vi "Begin.vi"() -> (0 "error out":errorcluster)   [LabVIEW 2013]
doc: "Called before other user functions, this VI is expected to open initial I/O refnums, load in file data, and do all program initialization. Notice that the <B>error out</B> terminal is simply used for data flow. Wiring it to other structures or subVIs ensures that this VI runs first."
uses:
  <vilib>/Rock Robotics/WPI/SafetyOutput/WPI_SafetyOutputConfigMenu.ctl
  <vilib>/Rock Robotics/WPI/DriverStation/WPI_DriverStationRobotMode2.ctl
  <vilib>/Rock Robotics/WPI/Joystick/WPI_JoystickDeviceEnum.ctl
  <vilib>/Rock Robotics/SystemInterfaces/DIO/FPGA_DIOPWMChannel.ctl
  <vilib>/Rock Robotics/SystemInterfaces/DIO/FPGA_DIOChannel.ctl
  <vilib>/Rock Robotics/SystemInterfaces/DIO/FPGA_DIORelayChannel.ctl
  <vilib>/Rock Robotics/SystemInterfaces/Typedef/FPGA_TypedefDigitalModule.ctl
  <vilib>/Rock Robotics/WPI/Camera/WPI_CameraImageSize.ctl
  <vilib>/Rock Robotics/WPI/Camera/WPI_CameraFrameRate.ctl
  <vilib>/Rock Robotics/WPI/Camera/WPI_CameraWhite Balance Values.ctl
  <vilib>/Rock Robotics/WPI/Camera/WPI_CameraExposure Values.ctl
  <vilib>/Rock Robotics/WPI/Solenoid/WPI_SolenoidChannel.ctl
  <vilib>/Rock Robotics/SystemInterfaces/AI/FPGA_AIChannel.ctl
  <vilib>/Rock Robotics/SystemInterfaces/Typedef/FPGA_TypedefAnalogModule.ctl
  Robot Global Data.vi
  <vilib>/Rock Robotics/WPI/MotorControl/WPI_MotorControlOpen Talon.vi
  <vilib>/Rock Robotics/WPI/Solenoid/WPI_SolenoidOpenDouble.vi
  <vilib>/Rock Robotics/WPI/RobotDrive/WPI_RobotDriveOpen4MotorWithTalon.vi
  <vilib>/Rock Robotics/WPI/Compressor/WPI_CompressorGetSetRefNum.vi
panel:
  out "Boolean Array":bool[](array[boolean])
  in  "Dashbord/Constant":bool
  out "error out 3":errorcluster
  out "error out 2":errorcluster
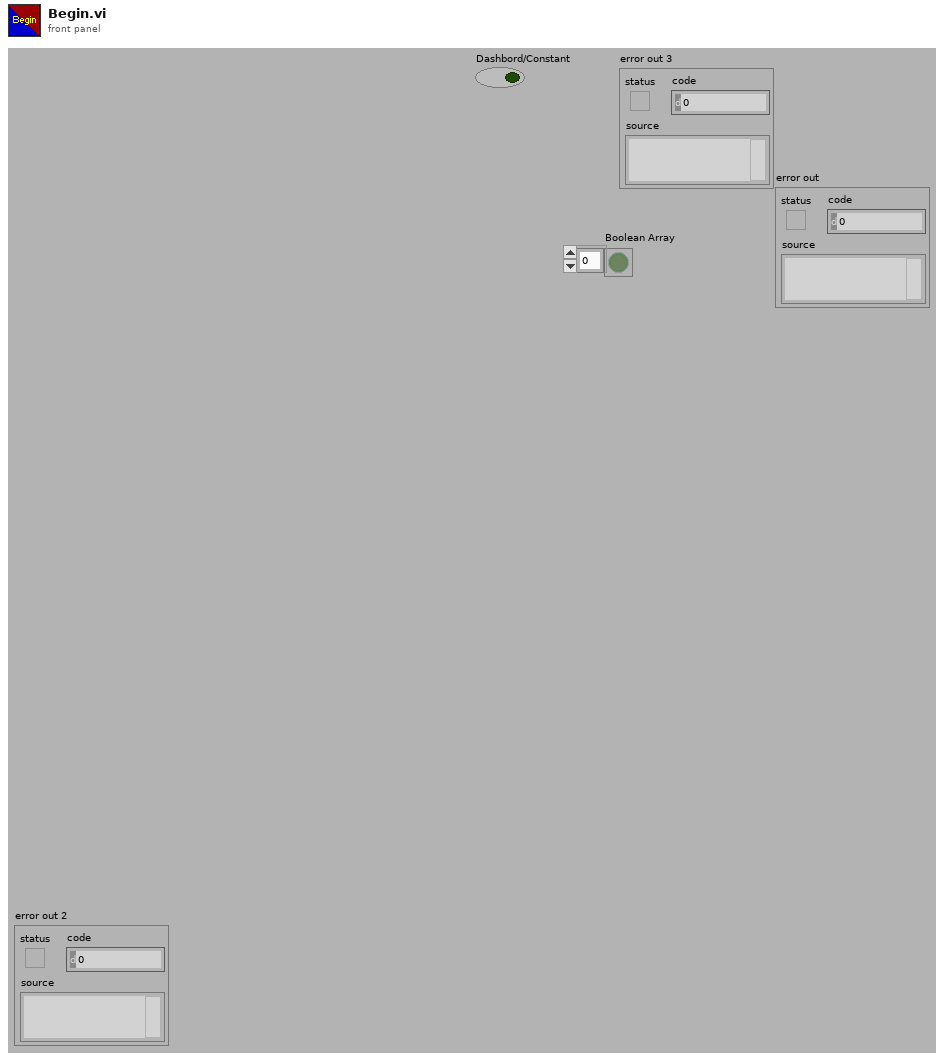
[diagram p1: front panel]
types:
  T1 = typedef "FPGA_TypedefAnalogModule.ctl" = enum16{"Analog Module 1", "Analog Module 2"}
  T2 = typedef "FPGA_AIChannel.ctl" = enum8{"AI 1", "AI 2", "AI 3", "AI 4", "AI 5", "AI 6", "AI 7", "AI 8", "Invalid"}
  T3 = typedef "WPI_SolenoidChannel.ctl" = enum8{"Solenoid 1", "Solenoid 2", "Solenoid 3", "Solenoid 4", "Solenoid 5", "Solenoid 6", "Solenoid 7", "Solenoid 8", "Invalid"}
  T4 = typedef "FPGA_TypedefDigitalModule.ctl" = enum16{"Digital Module 1", "Digital Module 2"}
  T5 = typedef "WPI_CameraExposure Values.ctl" = enum16{"Auto", "Flicker-free 50 Hz", "Flicker-free 60 Hz", "Hold current"}
  T6 = typedef "WPI_CameraWhite Balance Values.ctl" = enum16{"Auto", "Fixed indoor", "Fixed outdoor 1", "Fixed outdoor 2", "Fixed fluorescent 1", "Fixed fluorescent 2", "Hold current"}
  T7 = typedef "WPI_CameraFrameRate.ctl" = u32
  T8 = typedef "WPI_CameraImageSize.ctl" = enum16{"640x480", "320x240", "160x120"}
  T9 = typedef "FPGA_DIOChannel.ctl" = enum8{"DIO 1", "DIO 2", "DIO 3", "DIO 4", "DIO 5", "DIO 6", "DIO 7", "DIO 8", "DIO 9", "DIO 10", "DIO 11", "DIO 12", "DIO 13", "DIO 14", "Invalid"}
  T10 = typedef "FPGA_DIORelayChannel.ctl" = enum8{"Relay 1", "Relay 2", "Relay 3", "Relay 4", "Relay 5", "Relay 6", "Relay 7", "Relay 8", "Invalid"}
  T11 = typedef "WPI_JoystickDeviceEnum.ctl" = enum16{"USB 1", "USB 2", "USB 3", "USB 4", "Kinect 1", "Kinect 2"}
  T12 = typedef "FPGA_DIOPWMChannel.ctl" = enum8{"PWM 1", "PWM 2", "PWM 3", "PWM 4", "PWM 5", "PWM 6", "PWM 7", "PWM 8", "PWM 9", "PWM 10", "Invalid"}
  T13 = typedef "WPI_DriverStationRobotMode2.ctl" = enum16{"Autonomous Disabled", "Autonomous Enabled", "Teleop Disabled", "Teleop Enabled", "Timeout", "Finish", "Test Disabled", "Test Enabled"}
  T14 = typedef "WPI_SafetyOutputConfigMenu.ctl" = enum16{"Enable", "Disable"}
  T15 = cluster{"Boolean Array[0]":bool, "Boolean Array[1]":bool, "Boolean Array[2]":bool, "Boolean Array[3]":bool, "Boolean Array[4]":bool, "Boolean Array[5]":bool, "Boolean Array[6]":bool, "Boolean Array[7]":bool, "Boolean Array[8]":bool}
  T16 = typedef "WPI_MotorControlDeviceRef.ctl" = cluster{"DeviceStatus":errorcluster, "Type":enum16{"PWM", "CAN"}, "PWM":cluster{"Digital Module":T4, "PWM Channel":T12, "DeadBand":T17}, "CAN":cluster{"Device Number":u8, "Control Mode":T18, "Semaphore":T19, "Max Vout":dbl}, "Invert":bool, "TransformRef":T20, "InvTransformRef":T20}
  T17 = typedef "WPI_PWMDeadband.ctl" = cluster{"Name":string, "maxPositivePwm":i32, "minPositivePwm":i32, "centerPwm":i32, "maxNegativePwm":i32, "minNegativePwm":i32, "angularRange":u16}
  T18 = typedef "WPI_CANJaguar_ControlMode.ctl" = enum8{"Percent VBus", "Current", "Speed", "Position", "Voltage"}
  T19 = typedef "Semaphore RefNum" = refnum<k1>
  T20 = typedef "WPI_PWMTransform_ConPane.ctl" = refnum<vi>
  T21 = typedef "WPI_RobotDriveDevRef.ctl" = cluster{"DevStatus":errorcluster, "Motors[]":T16[], "Square Inputs":bool, "Max Output":dbl, "Isochronous":bool}
  T22 = typedef "WPI_CompressorDevRef.ctl" = cluster{"DevStatus":errorcluster, "DigitalInputDevRef":T23, "RelayDevRef":T24}
  T23 = typedef "WPI_DigitalInputDevRef.ctl" = cluster{"DevStatus":errorcluster, "DIO Channel":T9, "Digital Module":T4}
  T24 = typedef "WPI_RelayDevRef.ctl" = cluster{"DevStatus":errorcluster, "Relay Channel":T10, "Digital Module":T4, "Relay Direction":T25}
  T25 = typedef "WPI_RelayDirection.ctl" = enum16{"Both directions", "Forward only", "Reverse only"}
  T26 = typedef "WPI_CameraDevRef.ctl" = cluster{"Camera Address":string, "CameraStatus":errorcluster, "Acquire Image Notifier":refnum<notifier>}
  T27 = typedef "WPI_SolenoidDevRef.ctl" = cluster{"DevStatus":errorcluster, "Solenoid Module":T28, "Forward Solenoid Channel":T3, "Reverse Solenoid Channel":T3}
  T28 = typedef "FPGA_TypedefSolenoidModule.ctl" = enum16{"Solenoid Module 1", "Solenoid Module 2"}
  T29 = typedef "WPI_JoystickDevRef.ctl" = cluster{"Device":T11}
  T30 = typedef "WPI_UltrasonicDeviceRef.ctl" = cluster{"DevStatus":errorcluster, "Ping Digital Module":T4, "Echo Digital Module":T4, "Ping Channel":T9, "Echo Channel":T9, "CntIndex":T31}
  T31 = typedef "FPGA_CounterCtrSystemIndex.ctl" = enum8{"Ctr 0", "Ctr 1", "Ctr 2", "Ctr 3", "Ctr 4", "Ctr 5", "Ctr 6", "Ctr 7", "Invalid"}
  T32 = typedef "WPI_AnalogChannelDevRef.ctl" = cluster{"DevStatus":errorcluster, "Analog Module":T1, "Analog Channel":T2}
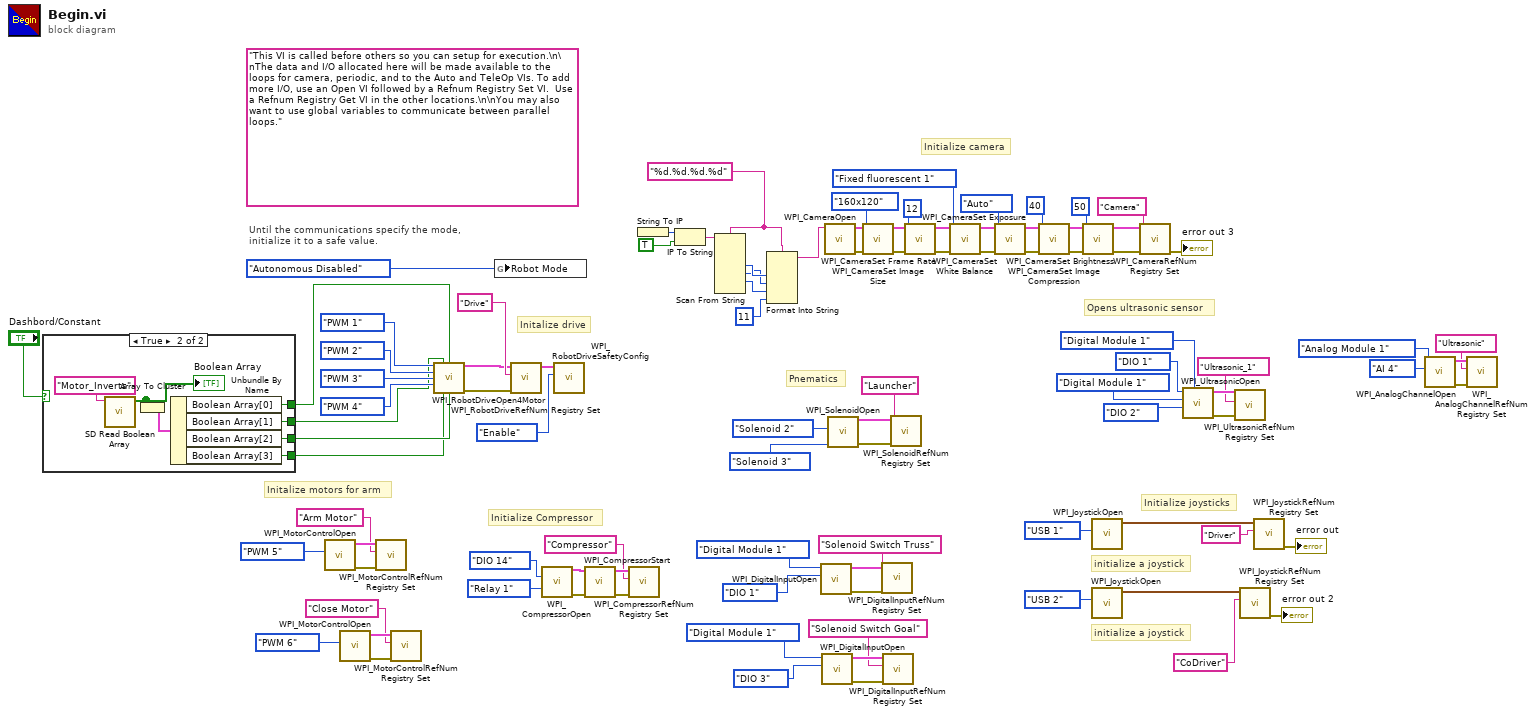
[diagram p0: block diagram]
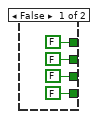
[diagram p2: hidden frame]
diagram:
  w23 = "%d.%d.%d.%d" ("Camera Address")
  (unwired) "This VI is called before others so you can setup for execution.\n\nThe data and I/O allocated here will be made available to the loops for camera, periodic, and to the Auto and TeleOp VIs. To add more I/O, use an Open VI followed by a Refnum Registry Set VI.  Use a Refnum Registry Get VI in the other locations.\n\nYou may also want to use global variables to communicate between parallel loops."
  # "Pnematics"
  # "Opens ultrasonic sensor"
  # "Initialize Compressor"
  # "Initalize motors for arm"
  # "Initialize camera"
  # "Initialize joysticks"
  # "initialize a joystick"
  # "initialize a joystick"
  # "Until the communications specify the mode,\ninitialize it to a safe value."
  # "Initalize drive"
  n1 = case shown="True" "Dashbord/Constant" {
    tunnel: [FALSE ("Boolean Array[0]") w104] -> w5
    tunnel: [FALSE ("Boolean Array[1]") w103] -> w4
    tunnel: [FALSE ("Boolean Array[2]") w102] -> w3
    tunnel: [FALSE ("Boolean Array[3]") w101] -> w2
    frame False {
    }
    frame True {
      n2 = call <vilib>:"SD Read Boolean Array.vi"("Name"="Motor_Inverts") -> ("Boolean Array"=w106:bool[])  [unwired: 8 in, 2 out]
      "Boolean Array" <- w106
      n3 = Array To Cluster(array=w106) -> (cluster=w105:T15)
      n4 = Unbundle By Name(w105) -> ("Boolean Array[0]"=w104:bool, "Boolean Array[1]"=w103:bool, "Boolean Array[2]"=w102:bool, "Boolean Array[3]"=w101:bool)
    }
  }
  n5 = call-poly <vilib>:"WPI_MotorControlOpen.vi"("PWM Channel"=FPGA_DIOPWMChannel."PWM 5") -> ("error out"=w79:errorcluster, "MotorControlDeviceRef"=w80:T16)  [unwired: 9 in]
  n6 = call-poly <vilib>:"WPI_MotorControlOpen.vi"("PWM Channel"=FPGA_DIOPWMChannel."PWM 6") -> ("error out"=w77:errorcluster, "MotorControlDeviceRef"=w78:T16)  [unwired: 9 in]
  n7 = call <vilib>:"WPI_MotorControlRefNum Registry Set.vi"("error in (no error)"=w79, "refnum name"="Arm Motor", "MotorControlDevRef"=w80) -> ()  [unwired: 7 in, 2 out]
  n8 = call <vilib>:"WPI_MotorControlRefNum Registry Set.vi"("error in (no error)"=w77, "refnum name"="Close Motor", "MotorControlDevRef"=w78) -> ()  [unwired: 7 in, 2 out]
  n9 = call-poly <vilib>:"WPI_RobotDriveOpen4Motor.vi"("Rear Left Motor"=FPGA_DIOPWMChannel."PWM 1", "Rear Left Motor Inverted"=w4, "Rear Right Motor Inverted"=w5, "Rear Right Motor"=FPGA_DIOPWMChannel."PWM 2", "Front Left Motor"=FPGA_DIOPWMChannel."PWM 3", "Front Right Motor"=FPGA_DIOPWMChannel."PWM 4", "Front Left Motor Inverted"=w2, "Front Right Motor Inverted"=w3) -> ("RobotDriveDevRef"=w88:T21, "error out"=w87:errorcluster)  [unwired: 6 in]
  n10 = global write "Robot Global Data.vi" "Robot Mode"(WPI_DriverStationRobotMode2."Autonomous Disabled" ("Robot Mode")) -> ()
  n11 = call <vilib>:"WPI_RobotDriveRefNum Registry Set.vi"("error in (no error)"=w87, "refnum name"="Drive", "RobotDriveDevRef"=w88) -> ("RobotDriveDevRef"=w95:T21)  [unwired: 8 out]
  n12 = call <vilib>:"WPI_CompressorOpen.vi"("Pressure Switch DIO Channel"=FPGA_DIOChannel."DIO 14", "Relay Channel"=FPGA_DIORelayChannel."Relay 1") -> ("CompressorDevRef"=w68:T22, "error out"=w67:errorcluster)  [unwired: 12 in]
  n13 = call <vilib>:"WPI_RobotDriveSafetyConfig.vi"("mode"=WPI_SafetyOutputConfigMenu."Enable", "RobotDriveDevRef"=w95) -> ()  [unwired: 8 in, 2 out]
  n14 = call <vilib>:"WPI_CompressorStart.vi"("error in (no error)"=w67, "CompressorDevRef"=w68) -> ("error out"=w65:errorcluster, "CompressorDevRef"=w66:T22)  [unwired: 8 in]
  n15 = call <vilib>:"WPI_CompressorRefNum Registry Set.vi"("error in (no error)"=w65, "refnum name"="Compressor", "CompressorDevRef"=w66) -> ()  [unwired: 7 in, 2 out]
  n16 = String To IP() -> (0:w25:u32)  [unwired: 1 in]
  n17 = IP To String(1:TRUE ("dot notation? (F)"), 2:w25) -> (0:w24:string)
  n18 = Scan From String(format string=w23, input string=w24) -> (output 1=w22:i32, output 2=w20:i32, output 3=w19:i32)  [unwired: 7 in, 3 out]
  n19 = Format Into String(format string=w23, w22, w20, w19, 11) -> (resulting string=w21:string)  [unwired: 2 in, 1 out]
  n20 = call <vilib>:"WPI_DigitalInputOpen.vi"("DIO Channel"=FPGA_DIOChannel."DIO 1", "Digital Module (Module 1)"=FPGA_TypedefDigitalModule."Digital Module 1") -> ("error out"=w63:errorcluster, "DigitalInputDevRef"=w62:T23)  [unwired: 8 in]
  n21 = call <vilib>:"WPI_DigitalInputOpen.vi"("DIO Channel"=FPGA_DIOChannel."DIO 3", "Digital Module (Module 1)"=FPGA_TypedefDigitalModule."Digital Module 1") -> ("error out"=w61:errorcluster, "DigitalInputDevRef"=w60:T23)  [unwired: 8 in]
  n22 = call <vilib>:"WPI_CameraOpen.vi"("Camera Address"=w21) -> ("error out"=w47:errorcluster, "CameraDevRef"=w46:T26)  [unwired: 9 in]
  n23 = call-poly <vilib>:"WPI_SolenoidOpen.vi"("Reverse Solenoid Channel"=WPI_SolenoidChannel."Solenoid 3", "Forward Solenoid Channel"=WPI_SolenoidChannel."Solenoid 2") -> ("error out"=w12:errorcluster, "SolenoidDevRef"=w13:T27)  [unwired: 8 in]
  n24 = call <vilib>:"WPI_CameraSet Image Size.vi"("error in (no error)"=w47, "Image Size"=WPI_CameraImageSize."160x120", "CameraDevRef"=w46) -> ("error out"=w44:errorcluster, "CameraDevRef Out"=w43:T26)  [unwired: 7 in]
  n25 = call <vilib>:"WPI_DigitalInputRefNum Registry Set.vi"("error in (no error)"=w63, "refnum name"="Solenoid Switch Truss", "DigitalInputDevRef"=w62) -> ()  [unwired: 7 in, 2 out]
  n26 = call <vilib>:"WPI_DigitalInputRefNum Registry Set.vi"("error in (no error)"=w61, "refnum name"="Solenoid Switch Goal", "DigitalInputDevRef"=w60) -> ()  [unwired: 7 in, 2 out]
  n27 = call <vilib>:"WPI_SolenoidRefNum Registry Set.vi"("error in (no error)"=w12, "refnum name"="Launcher", "SolenoidDevRef"=w13) -> ()  [unwired: 7 in, 2 out]
  n28 = call <vilib>:"WPI_CameraSet Frame Rate.vi"("error in (no error)"=w44, "Frame Rate (fps)"=T7 12, "CameraDevRef"=w43) -> ("error out"=w41:errorcluster, "CameraDevRef Out"=w40:T26)  [unwired: 7 in]
  n29 = call <vilib>:"WPI_CameraSet White Balance.vi"("error in (no error)"=w41, "White Balance"=WPI_CameraWhite_Balance_Values."Fixed fluorescent 1", "CameraDevRef"=w40) -> ("error out"=w38:errorcluster, "CameraDevRef Out"=w37:T26)  [unwired: 7 in]
  n30 = call <vilib>:"WPI_CameraSet Exposure.vi"("error in (no error)"=w38, "Exposure"=WPI_CameraExposure_Values."Auto", "CameraDevRef"=w37) -> ("error out"=w35:errorcluster, "CameraDevRef Out"=w34:T26)  [unwired: 7 in]
  n31 = call <vilib>:"WPI_CameraSet Image Compression.vi"("error in (no error)"=w35, "Compression"=40, "CameraDevRef"=w34) -> ("error out"=w32:errorcluster, "CameraDevRef Out"=w31:T26)  [unwired: 7 in]
  n32 = call <vilib>:"WPI_CameraSet Brightness.vi"("error in (no error)"=w32, "Brightness"=50, "CameraDevRef"=w31) -> ("error out"=w29:errorcluster, "CameraDevRef Out"=w28:T26)  [unwired: 7 in]
  n33 = call <vilib>:"WPI_JoystickOpen.vi"("JoystickDevice"=WPI_JoystickDeviceEnum."USB 1") -> ("JoystickDevRef"=w91:T29)  [unwired: 10 in]
  n34 = call <vilib>:"WPI_JoystickOpen.vi"("JoystickDevice"=WPI_JoystickDeviceEnum."USB 2") -> ("JoystickDevRef"=w73:T29)  [unwired: 10 in]
  n35 = call <vilib>:"WPI_CameraRefNum Registry Set.vi"("error in (no error)"=w29, "refnum name"="Camera", "CameraDevRef"=w28) -> ("error out"=→"error out 3":errorcluster)  [unwired: 7 in, 1 out]
  n36 = call <vilib>:"WPI_UltrasonicOpen.vi"("Ping Digital Module (Module 1)"=FPGA_TypedefDigitalModule."Digital Module 1", "Echo DIO Channel"=FPGA_DIOChannel."DIO 2", "Echo Digital Module (Module 1)"=FPGA_TypedefDigitalModule."Digital Module 1", "Ping DIO Channel"=FPGA_DIOChannel."DIO 1") -> ("error out"=w53:errorcluster, "UltrasonicDevRef"=w52:T30)  [unwired: 6 in]
  n37 = call <vilib>:"WPI_UltrasonicRefNum Registry Set.vi"("error in (no error)"=w53, "refnum name"="Ultrasonic_1", "UltrasonicDevRef"=w52) -> ()  [unwired: 7 in, 2 out]
  n38 = call <vilib>:"WPI_JoystickRefNum Registry Set.vi"("refnum name"="CoDriver", "JoystickDevRef"=w73) -> ("error out"=→"error out 2":errorcluster)  [unwired: 8 in, 1 out]
  n39 = call <vilib>:"WPI_JoystickRefNum Registry Set.vi"("refnum name"="Driver", "JoystickDevRef"=w91) -> ("error out"=→"error out":errorcluster)  [unwired: 8 in, 1 out]
  n40 = call <vilib>:"WPI_AnalogChannelOpen.vi"("Analog Channel"=FPGA_AIChannel."AI 4", "Analog Module (Module 1)"=FPGA_TypedefAnalogModule."Analog Module 1") -> ("error out"=w8:errorcluster, "AIDeviceRef"=w7:T32)  [unwired: 8 in]
  n41 = call <vilib>:"WPI_AnalogChannelRefNum Registry Set.vi"("error in (no error)"=w8, "refnum name"="Ultrasonic", "AIDeviceRef"=w7) -> ()  [unwired: 7 in, 2 out]
